vi "DEPP Stream.vi"() -> ()   [LabVIEW 2011, in "LVH-Adept.lvlib"]
uses:
  LVH-Adept.lvlib
  Private/DMGR/DMGR.lvlib
  Private/DEPP/DEPP.lvlib
panel:
  in  "Data 2":u8
  out "Data":u8[](array[numeric])
  in  "Num Bytes":u8
  in  "Address":u8
  out "Error Out":errorcluster
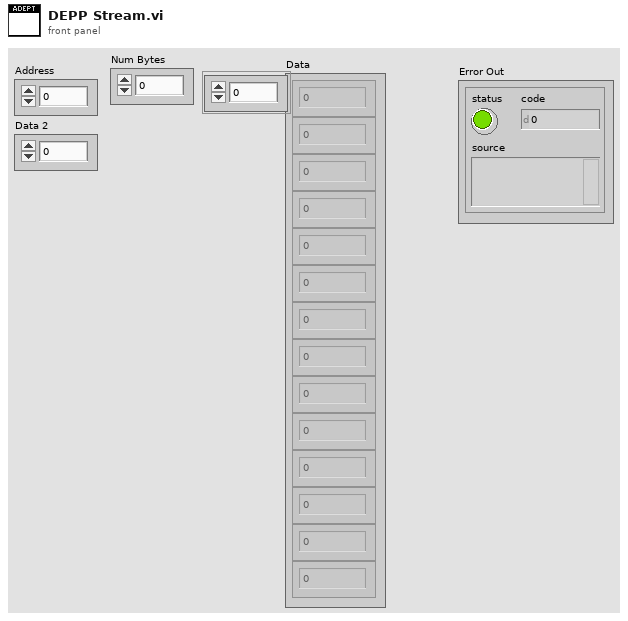
[diagram p1: front panel]
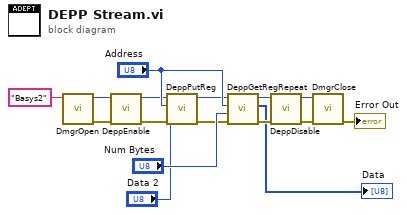
[diagram p0: block diagram]
diagram:
  n1 = call "DmgrOpen.vi"("Device Name"="Basys2") -> ("Error Out"=w16:errorcluster, "Device Handle"=w13:u32)  [unwired: 9 in]
  n2 = call "DeppEnable.vi"("Error In"=w16, "Device Handle"=w13) -> ("Error Out"=w8:errorcluster, "Device Handle"=w5:u32)  [unwired: 8 in]
  n3 = call "DeppPutReg.vi"("Error In"=w8, "Data"="Data 2", "Address"="Address", "Device Handle"=w5) -> ("Error Out"=w7:errorcluster, "Device Handle"=w4:u32)  [unwired: 6 in]
  n4 = call "DeppGetRegRepeat.vi"("Error In"=w7, "Num Bytes"="Num Bytes", "Address"="Address", "Device Handle"=w4) -> ("Error Out"=w6:errorcluster, "Data"=→"Data":u8[], "Device Handle"=w3:u32)  [unwired: 5 in]
  n5 = call "DeppDisable.vi"("Error In"=w6, "Device Handle"=w3) -> ("Error Out"=w15:errorcluster, "Device Handle"=w14:u32)  [unwired: 8 in]
  n6 = call "DmgrClose.vi"("Error In"=w15, "hif"=w14) -> ("Error Out"=→"Error Out":errorcluster)  [unwired: 9 in]
